vi "Format Image Structure.vi"(4 "Max Height (50 pixels)":i16=50, 6 "Max Width (500 pixels)":i16=500, 8 "error in (no error)":errorcluster {"code" format="Error %.0f"}, 10 "Image":path, 11 "VIDoc Printer - Confluence In":refnum<class "VIDoc Printer - Confluence.lvclass">) -> (0 "error out":errorcluster {"code" format="Error %.0f"}, 2 "Image Structure Text":string, 3 "VIDoc Printer - Confluence Out":refnum<class "VIDoc Printer - Confluence.lvclass">)   [LabVIEW 2023, in "VIDoc Printer - Confluence.lvlib" / "VIDoc Printer - Confluence.lvclass"]
uses:
  VIDoc Printer - Confluence.lvclass
  VIDoc Printer - Confluence.lvclass/VIDoc Printer - Confluence.ctl
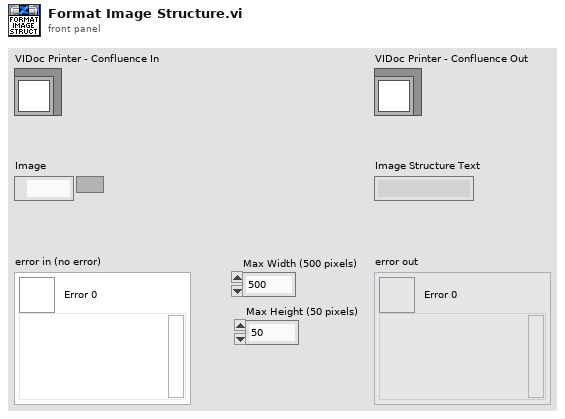
[diagram p1: front panel]
types:
  T1 = typedef "imagedata.ctl" = cluster{"image type":i32, "image depth":i32, "image":u8[], "mask":u8[], "colors":u32[], "Rectangle":cluster{"left":i16, "top":i16, "right":i16, "bottom":i16}}
  T2 = cluster{"left":i16, "top":i16, "right":i16, "bottom":i16}
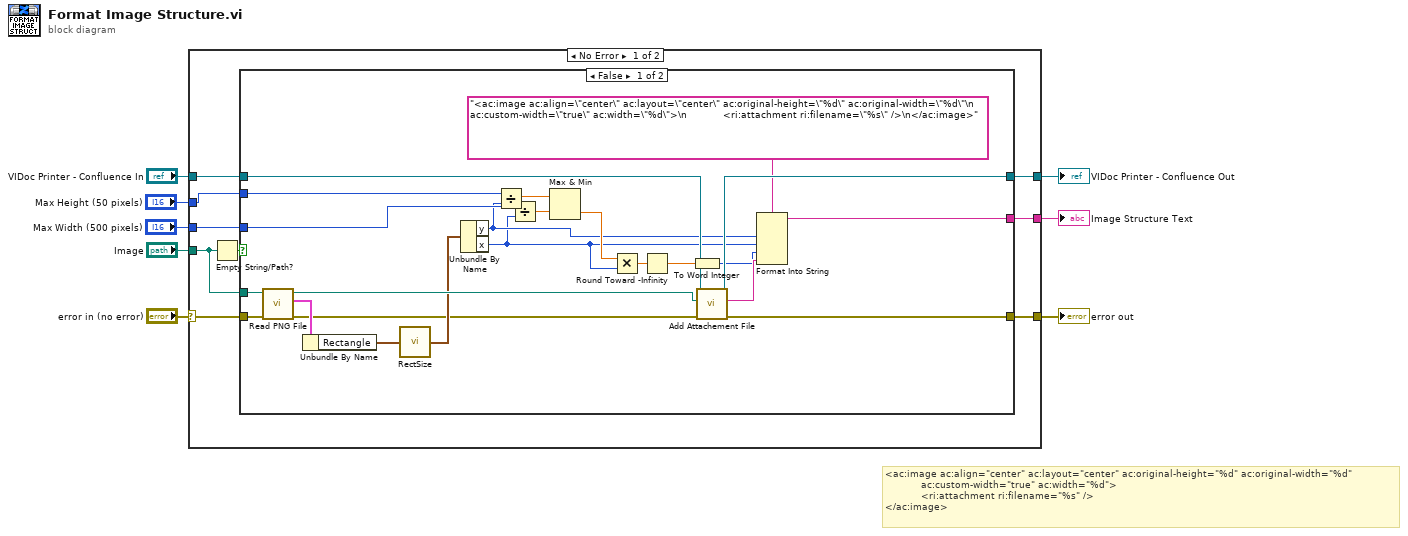
[diagram p0: block diagram]
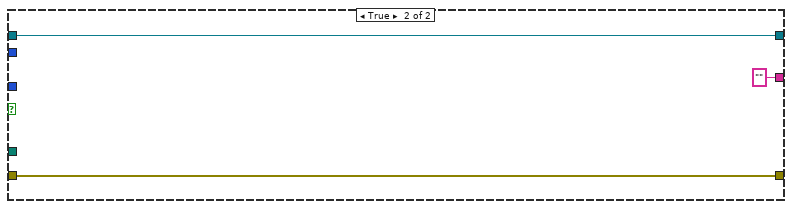
[diagram p2: hidden frame]
diagram:
  # "<ac:image ac:align=\"center\" ac:layout=\"center\" ac:original-height=\"%d\" ac:original-width=\"%d\"\n            ac:custom-width=\"true\" ac:width=\"%d\">\n            <ri:attachment ri:filename=\"%s\" />\n</ac:image>"
  n1 = case shown="No Error" "error in (no error)" {
    selector: "error in (no error)" -> [w13 w45]
    tunnel: [w15 w45] -> w7
    tunnel: [w17 w44] -> w5
    tunnel: "VIDoc Printer - Confluence In" -> [w16 w44]
    tunnel: "Image" -> [w10 _]
    tunnel: [w14 _] -> w3
    tunnel: "Max Width (500 pixels)" -> [w11 _]
    tunnel: "Max Height (50 pixels)" -> [w12 _]
    frame No Error {
      n2 = Empty String/Path?(string/path=w10) -> (empty?=w9:bool)
      n3 = case shown="False" w9 {
        tunnel: [w40 w42] -> w17
        tunnel: w16 -> [w39 w42]
        tunnel: [w38 w43] -> w15
        tunnel: [w36 ""] -> w14
        tunnel: w10 -> [w35 _]
        tunnel: w13 -> [w34 w43]
        tunnel: w12 -> [w27 _]
        tunnel: w11 -> [w26 _]
        frame False {
          n4 = call <vilib>:"Read PNG File.vi"("error in (no error)"=w34, "path to PNG file"=w35) -> ("error out"=w28:errorcluster, "image data"=w32:T1, "path"=w33:path)  [unwired: 7 in]
          n5 = Unbundle By Name(w32) -> ("Rectangle"=w31:T2)
          n6 = call <vilib>:"RectSize.vi"("rect"=w31) -> ("point"=w30:cluster{"x":i16, "y":i16})
          n7 = Unbundle By Name(w30) -> ("y"=w21:i16, "x"=w20:i16)
          n8 = Divide(x=w27, y=w21) -> (x/y=w25:dbl)
          n9 = Divide(x=w26, y=w20) -> (x/y=w24:dbl)
          n10 = Max & Min(x=w25, y=w24) -> (min(x,y)=w23:dbl)  [unwired: 1 out]
          n11 = Multiply(x=w23, y=w20) -> (x*y=w22:dbl)
          n12 = Round Toward -Infinity(1:w22) -> (0:w19:dbl)
          n13 = To Word Integer(number=w19) -> (16bit integer=w18:i16)
          n14 = call "Add Attachement File.vi"("error in (no error)"=w28, "File"=w33, "VIDoc Printer - Confluence In"=w39) -> ("error out"=w38:errorcluster, "Attachement FileName"=w29:string, "VIDoc Printer - Confluence Out"=w40:refnum<class "VIDoc Printer - Confluence.lvclass">)  [unwired: 6 in]
          n15 = Format Into String(format string="<ac:image ac:align=\"center\" ac:layout=\"center\" ac:original-height=\"%d\" ac:original-width=\"%d\"\n            ac:custom-width=\"true\" ac:width=\"%d\">\n            <ri:attachment ri:filename=\"%s\" />\n</ac:image>", w21, w20, w18, w29) -> (resulting string=w36:string)  [unwired: 2 in, 1 out]
        }
        frame True {
        }
      }
    }
    frame Error {
    }
  }
  "error out" <- w7
  "VIDoc Printer - Confluence Out" <- w5
  "Image Structure Text" <- w3
